vi "CC FITS Write Filter Names.vi"(8 "error in (no error)":errorcluster, 11 "gfits refnum":T1) -> (0 "error out":errorcluster, 3 "dup gfits refnum":T1)   [LabVIEW 2024]
uses:
  gfitsio/gfitsio-refnum.ctl
  Logging/CC enum Current Values Action.ctl
  gfitsio/gfitsio-write-key-string.vi
  hk-channel-class/hk-channel-class/HK Table/HK Table.lvclass
  gfitsio/gfitsio.lvlib
  Filter Wheel/Filter Wheel Object/Filter Wheel.lvclass
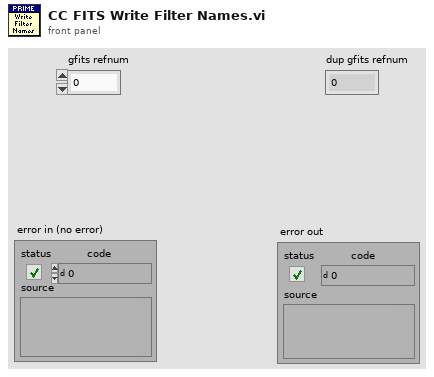
[diagram p1: front panel]
types:
  T1 = typedef "gfitsio.lvlib/gfitsio-refnum.ctl" = u64
  T2 = typedef "CC enum Current Values Action.ctl" = enum16{"Init", "Write Item", "Write Array", "Read Item", "Read Array", "Read All", "Add Channels", "New File", "Add Message", "Get Current Values", "Close"}
  T3 = typedef "Filter Wheel.lvclass/Filter Wheel configuration.ctl" = cluster{"Num Wheels":i32, "Filters":T4[], "Invalid Combinations":i32[][], "Addr":refnum<visa-resource-name>, "Name":string, "Simulate":bool, "Default Speed":u16, "Homing":T5[]}
  T4 = typedef "Filter Wheel.lvclass/Filter Wheel Details.ctl" = cluster{"Names":string[], "Relative Position":i32[], "Wheel Name":string, "Size":i32}
  T5 = typedef "Filter Wheel Arduino Homing cluster.ctl" = cluster{"Direction":bool, "Speed":i32, "Accel":i32, "Error Cnts":i32, "Homing Delta":i32}
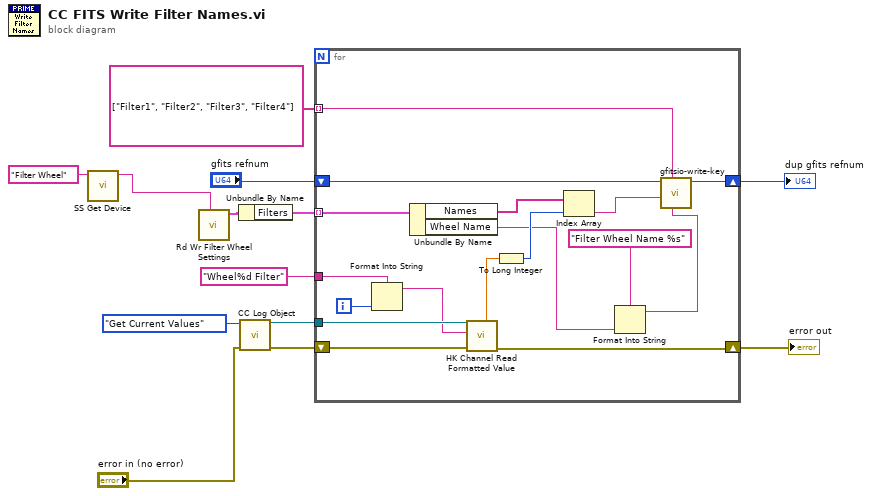
[diagram p0: block diagram]
diagram:
  n1 = call "SS Get Device.vi"("Device Type"="Filter Wheel") -> ("Device Name"=w2:string)  [unwired: 9 in, 1 out]
  n2 = call "Rd Wr Filter Wheel Settings.vi"("Wheel Name"=w2) -> ("Filter Wheel Settings"=w6:T3)  [unwired: 9 in, 1 out]
  n3 = Unbundle By Name(w6) -> ("Filters"=w5:T4[])
  n4 = call "CC Log Object.vi"("error in (no error)"="error in (no error)", "Action"=CC_enum_Current_Values_Action."Get Current Values") -> ("error out"=w8:errorcluster, "HK Channel out"=w12:refnum<class "HK Table.lvclass">)  [unwired: 7 in, 1 out]
  n5 = for {
    tunnel: w12 -> [w30]
    shift-right: [w28] -> w10
    shift-left: "gfits refnum" -> [w29]
    shift-right: [w26] -> w7
    shift-left: w8 -> [w27]
    tunnel: w5 -> [w24] mode=indexing
    tunnel: string[] ["Filter1", "Filter2", "Filter3", "Filter4"] -> [w20] mode=indexing
    tunnel: "Wheel%d Filter" ("format string") -> [w15]
    i -> [w16]
    n6 = Format Into String(format string=w15, w16) -> (resulting string=w14:string)  [unwired: 2 in, 1 out]
    n7 = Unbundle By Name(w24) -> ("Names"=w23:string[], "Wheel Name"=w18:string)
    n8 = call-dynamic "HK Channel Read Formatted Value.vi"("error in (no error)"=w27, "Name"=w14, "HK Table.lvclass"=w30) -> ("error out"=w26:errorcluster, "Value"=w25:dbl)  [unwired: 1 in, 6 out]
    n9 = To Long Integer(number=w25) -> (32bit integer=w22:i32)
    n10 = Index Array(array=w23, index=w22) -> (element=w21:string)
    n11 = Format Into String(format string="Filter Wheel Name %s", w18) -> (resulting string=w17:string)  [unwired: 2 in, 1 out]
    n12 = call-poly "gfitsio-write-key.vi"("comment"=w17, "keyname"=w20, "value"=w21, "gfits refnum"=w29) -> ("dup gfits refnum"=w28:T1)  [unwired: 6 in, 1 out]
  }
  "error out" <- w7
  "dup gfits refnum" <- w10
